vi "Keithley24XX_SR830_LakeShore336_I-Vg_Measurement.vi"() -> ()   [LabVIEW 2018]
uses:
  <instrlib>/Lake Shore 336/Public/Data/Sensor Data (Single Reading).vi
  <instrlib>/Stanford Research 830/Public/Data/Read (All Parameters).vi
  <instrlib>/Keithley 24XX/Public/Data/Read (Single Point).vi
  <instrlib>/Keithley 24XX/Keithley 24XX.lvlib
  <instrlib>/Stanford Research 830/Stanford Research 830.lvlib
  <instrlib>/Lake Shore 336/Lake Shore 336.lvlib
panel:
  in  "Loop Delay / Meas. Time (s)":dbl=1.0 format="%#_13g"
  out "Gate\nVoltage":sgl
  out "Status":sgl
  out "Leakage \nCurrent":sgl
  in  "Temp Vs Time":enum32{"XY Graph", "Waveform (Time)"}(tab)
  out "Temp vs Time : XYGraph":cluster{"Y":dbl[], "Y":dbl[]}[](graph)
  out "Temp vs Time : TimeGraph":cluster{i32, "Sensor Data":dbl}[](graph)
  in  "Data Source (0:Kelvin)":u16(ring) items=["Kelvin", "Celsius", "Sensor Units"]
  in  "Input (0:A)":u16(ring) items=["A", "B", "C", "D"]
  in  "Serial Configuration 2":T1={"Baud Rate"=57600, "Parity"=1, "Data Bits"=7, "Stop Bits"=10, "Flow Control"=0} {"Flow Control" items=["None", "XON/XOFF", "RTS/CTS", "XON/XOFF & RTS/CTS", "DTR/DSR", "XON/XOFF & DTR/DSR"]; "Stop Bits" items=["1.0"=10, "1.5"=15, "2.0"=20]; "Data Bits" items=["7"=7, "8"=8]; "Parity" items=["None", "Odd", "Even", "Mark", "Space"]; "Baud Rate" items=["300"=300, "600"=600, "1200"=1200, "2400"=2400, "4800"=4800, "9600"=9600, "19200"=19200, "38400"=38400, "57600"=57600]}
  in  "LakeShore 336 esource name":refnum<visa-resource-name>="GPIB0::12::INSTR"
  out "dup path":path
  in  "<File Name>.txt (Don't add extension)":string
  in  "Data Save Path:":path=path "C:/Users/labpc/Documents/ProbeStation Users Data"
  in  "I_leak vs Vg":enum32{"XY Graph", "Waveform (Time)"}(tab)
  out "I_leak vs Vg : XYGraph":cluster{"Y":dbl[], "Y":dbl[]}[](graph)
  out "I_leak vs Vg : TimeGraph":cluster{dbl, "Current":sgl}[](graph)
  in  "Gate Voltage\nInitial (V)":dbl
  out "Gate Voltage\nTraversal Direction":enum16{"Upward", "Downward"}(ring)
  in  "Gate Voltage \nStep Size (V)":dbl=0.1
  in  "High Gate \nVoltage (V)":dbl
  in  "Low Gate \nVoltage (V)":dbl
  in  "stop":bool
  out "Max/Min(-) \nGate Voltage (V)":dbl=80.0
  out "Compliance\n Level (A)":dbl=0.1
  in  "Theta vs Vg":enum32{"XY Graph", "Waveform (Time)"}(tab)
  out "Theta vs Vg : XYGraph":cluster{"Y":dbl[], "Y":dbl[]}[](graph)
  out "Theta vs Vg : TimeGraph":cluster{dbl, "Theta-Value":dbl}[](graph)
  in  "I vs Vg":enum32{"XY Graph", "Waveform (Time)"}(tab)
  out "Current vs Vg : XYGraph":cluster{"Y":dbl[], "Y":dbl[]}[](graph)
  out "I vs Vg : TimeGraph":cluster{dbl, dbl}[](graph)
  in  "Sensitivity (Initial Value)":i16(ring)=24 items=["Auto Gain"=-1, "2 nV/fA"=0, "5 nV/fA"=1, "10 nV/fA"=2, "20 nV/fA"=3, "50 nV/fA"=4, "100 nV/fA"=5, "200 nV/fA"=6, "500 nV/fA"=7, "1 uV/pA"=8, "2 uV/pA"=9, "5 uV/pA"=10, "10 uV/pA"=11, "20 uV/pA"=12, "50 uV/pA"=13, "100 uV/pA"=14, "200 uV/pA"=15, "500 uV/pA"=16, "1 mV/nA"=17, "2 mV/nA"=18, "5 mV/nA"=19, "10 mV/nA"=20, "20 mV/nA"=21, "50 mV/nA"=22, "100 mV/nA"=23, "200 mV/nA"=24, "500 mV/mA"=25, "1 V/uA"=26]
  in  "Dynamic Reserve (-1 = Auto)":i16(ring)=1 items=["Auto Reserve"=-1, "High Reserve"=0, "Normal"=1, "Low Noise"=2]
  in  "Input Connection (0: Single-Ended Voltage)":u16(ring)=2 items=["Single-Ended Voltage", "Differential Voltage", "1 MOhm Current Gain", "100 MOhm Current Gain"]
  out "Input Coupling (0: AC)":u16(ring) items=["AC", "DC"]
  in  "Time Constant (8: 100ms)":u16(ring)=9 items=["10 us", "30 us", "100 us", "300 us", "1 ms", "3 ms", "10 ms", "30 ms", "100 ms", "300 ms", "1 s", "3 s", "10 s", "30 s", "100 s", "300 s", "1 ks", "3 ks", "10 ks", "30 ks"]
  in  "SR830 VISA resource name":refnum<visa-resource-name>="GPIB0::10::INSTR"
  in  "Trigger Source (0: Internal)":u16(ring) items=["Internal", "External"]
  out "Manual Phase (0 Degree)":dbl
  out "Detection Harmonic Number":dbl=1.0
  out "External Reference Trigger (0: Sine Zero Crossing)":u16(ring) items=["Sine Zero Crossing", "TTL Rising Edge", "TTL Falling Edge"]
  in  "Internal Reference Frequency (1000 Hz)":dbl=7.6
  in  "Reference Source (1: Internal)":u16(ring)=1 items=["External", "Internal"]
  in  "Sine Output Amplitude (V)":dbl=1.0
  in  "Serial Configuration":T1={"Baud Rate"=9600, "Parity"=0, "Data Bits"=8, "Stop Bits"=10, "Flow Control"=0} {"Flow Control" items=["None", "XON/XOFF", "RTS/CTS", "XON/XOFF & RTS/CTS", "DTR/DSR", "XON/XOFF & DTR/DSR"]; "Stop Bits" items=["1.0"=10, "1.5"=15, "2.0"=20]; "Data Bits" items=["7"=7, "8"=8]; "Parity" items=["None", "Odd", "Even", "Mark", "Space"]; "Baud Rate" items=["300"=300, "600"=600, "1200"=1200, "2400"=2400, "4800"=4800, "9600"=9600, "19200"=19200]}
  in  "Keithley24XX VISA resource name":refnum<visa-resource-name>="GPIB0::21::INSTR" caption="Keithley 24XX VISA resource name"
  # "Lake Shore 336 Temp Contr."
  # "SR830 Lock In Amplifier"
  # "MAKE SURE THE SOURCE METER IS ON TO ENSURE NO UNINTENDED JUMPS. PROGRAM WILL KEEP SOURCE METER ON ONCE RUN."
  # "Keithley 2400 SourceMeter"
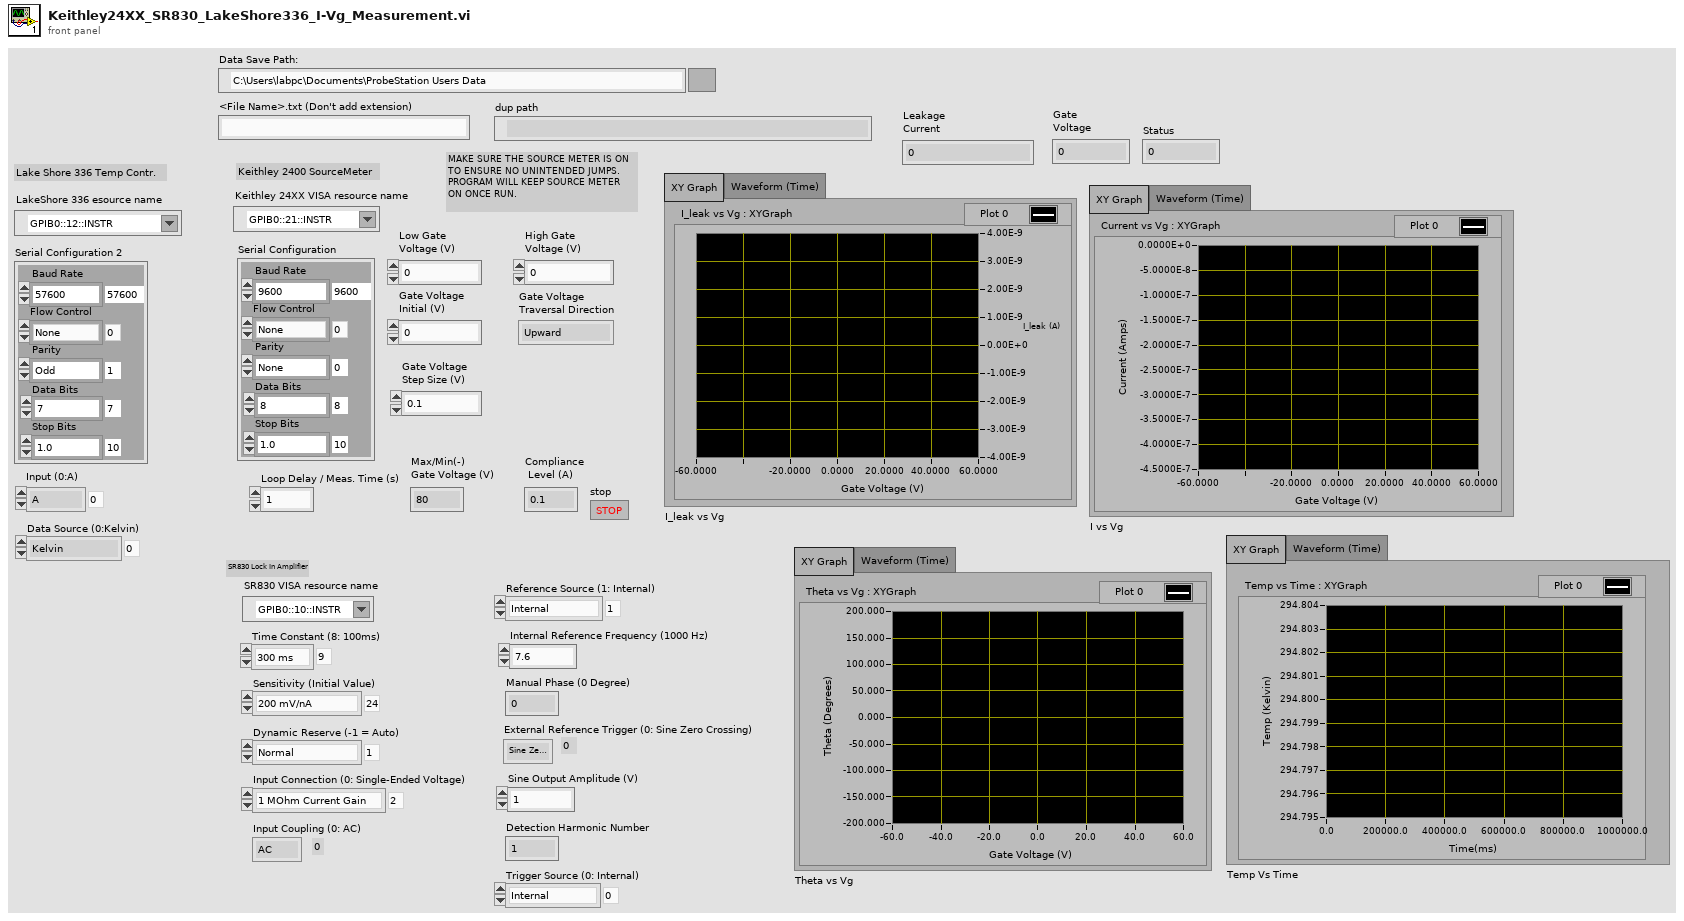
[diagram p1: front panel]
types:
  T1 = cluster{"Baud Rate":u32, "Parity":u16, "Data Bits":u16, "Stop Bits":u16, "Flow Control":u16}
  T2 = enum16{"open", "replace", "create", "open or create", "replace or create", "replace or create with confirmation"}
  T3 = cluster{"X-Value":dbl, "Y-Value":dbl, "R-Value":dbl, "Theta-Value":dbl, "Aux In 1 Value":dbl, "Aux In 2 Value":dbl, "Aux In 3 Value":dbl, "Aux In 4 Value":dbl, "Reference Frequency":dbl, "Channel 1 Display":dbl, "Channel 2 Display":dbl}
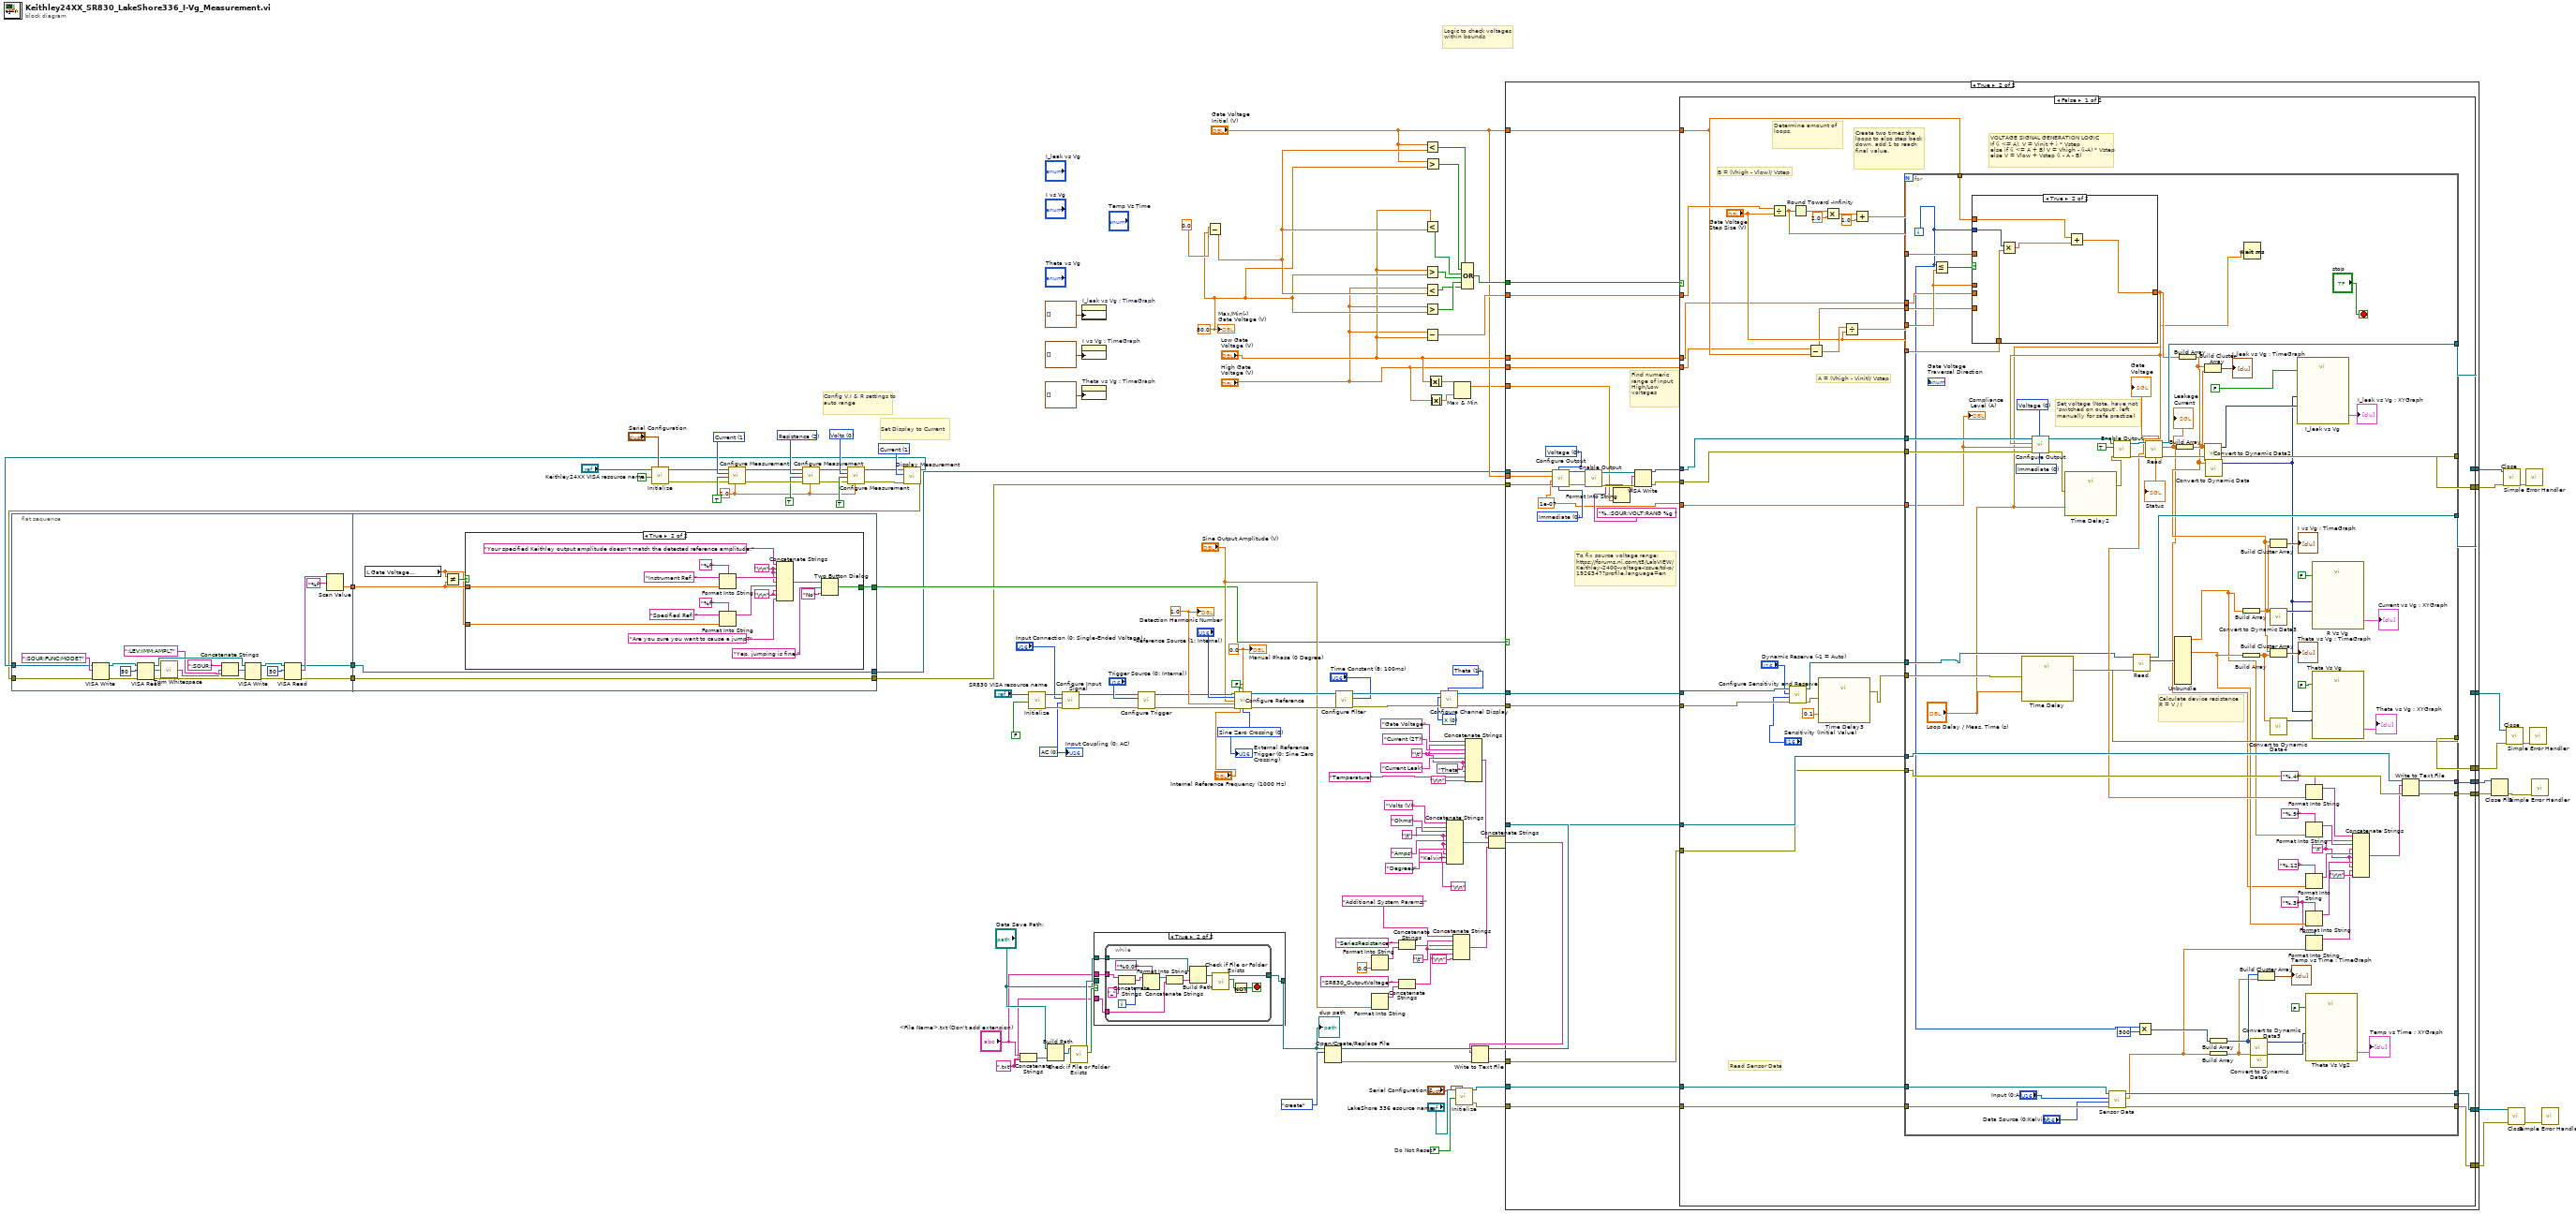
[diagram p0: block diagram]
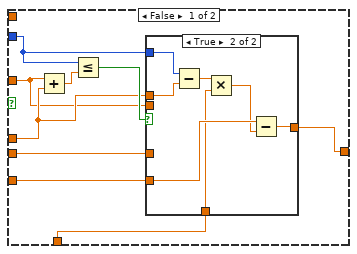
[diagram p3: hidden frame]
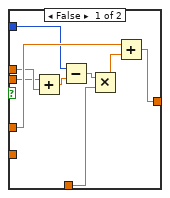
[diagram p4: hidden frame]
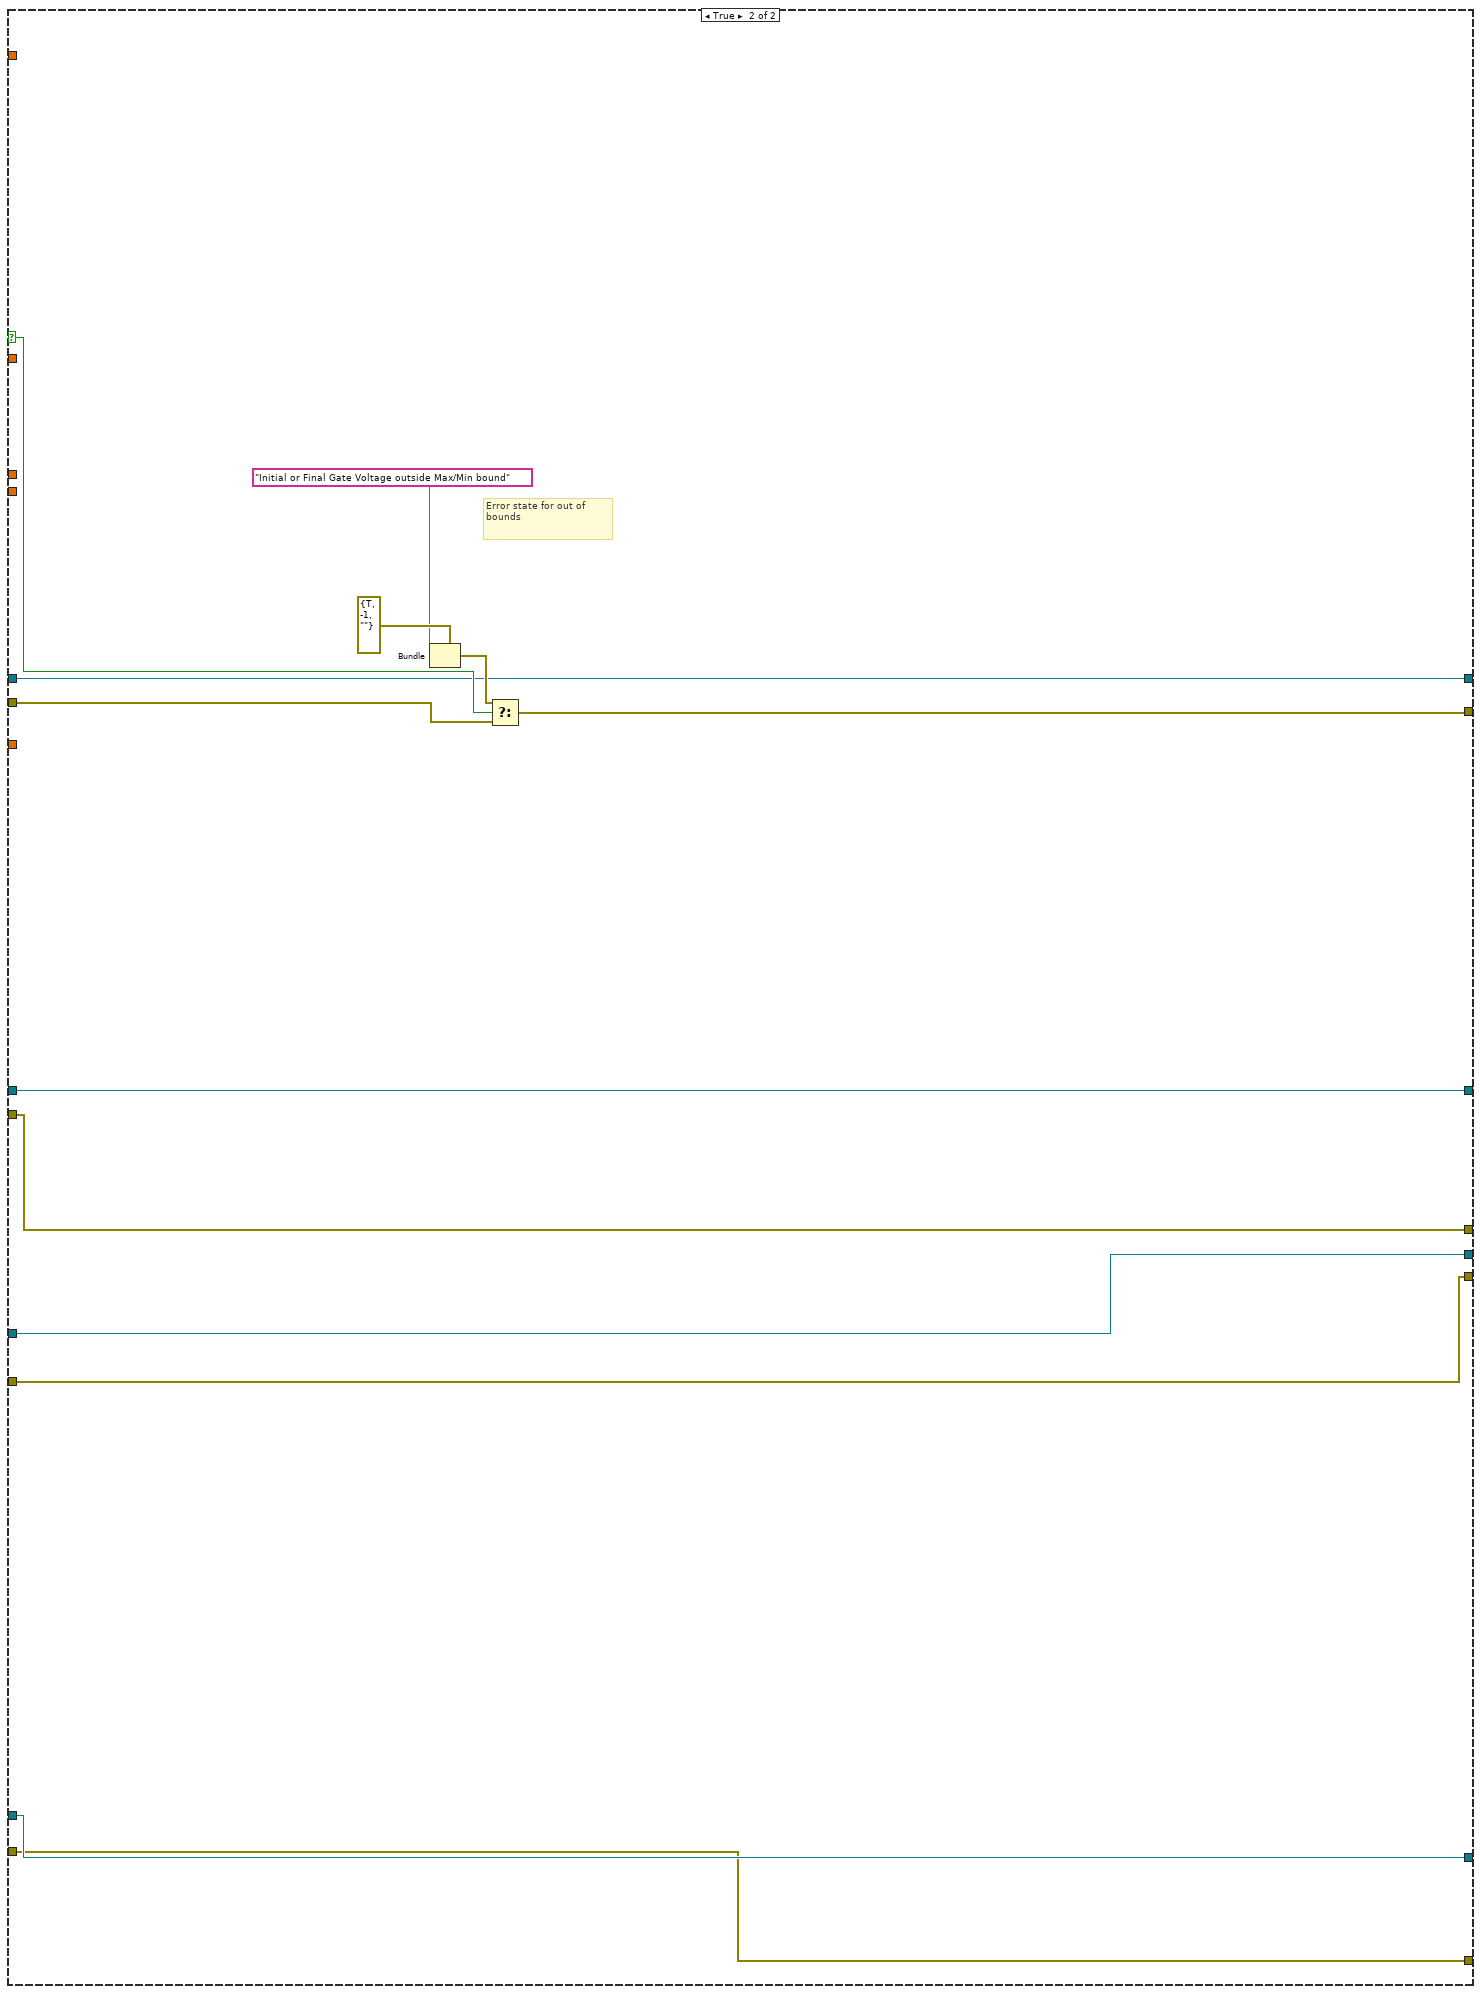
[diagram p5: hidden frame]
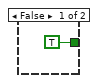
[diagram p6: hidden frame]
diagram:
  w28 = FALSE  # Do Not Reset
  w34 = "\t"
  w17 = "\t"
  w19 = "\t"
  w61 = ".txt"
  w68 = 1.0 ("Manual Range (1.0)")
  w91 = 0.0 ("Manual Phase (0 Degree)")
  w92 = 1.0 ("Detection Harmonic Number (1)")
  w93 = u16 0 items=["Sine Zero Crossing", "TTL Rising Edge", "TTL Falling Edge"] ("External Reference Trigger (0: Sine Zero Crossing)")
  w97 = u16 0 items=["AC", "DC"] ("Input Coupling (0: AC)")
  w80 = u16 0 items=["X", "R", "X Noise", "Aux In 1", "Aux In 2"] ("Channel 1 Display (0: X)")
  w107 = u16 1 items=["Y", "Theta", "Y Noise", "Aux In 3", "Aux In 4"] ("Channel 2 Display  (0: Y)")
  w112 = u16 1 items=["Voltage", "Current", "Resistance"] ("Displayed Measurement (0: Voltage)")
  w121 = u16 2 items=["Volts", "Current", "Resistance"] ("Function (0: Volts)")
  w125 = u16 1 items=["Volts", "Current", "Resistance"] ("Function (0: Volts)")
  w69 = 80.0
  w131 = u16 0 items=["Volts", "Current", "Resistance"] ("Function (0: Volts)")
  # "Logic to check voltages within bounds"
  # "Set Display to Current"
  # "Config V,I & R settings to auto range"
  n1 = flat-sequence {
    tunnel: [w135] -> w11
    tunnel: [w136] -> w10
    tunnel: [w137] -> w9
    tunnel: w8 -> [w134]
    tunnel: w7 -> [w133]
    tunnel: w11 -> [w156]
    tunnel: w10 -> [w155]
    tunnel: w9 -> [w159]
    tunnel: [w156] -> w3
    tunnel: [w155] -> w5
    tunnel: [w154] -> w6
    frame #0 {
      n2 = VISA Write(VISA resource name=w134, write buffer=":SOUR:FUNC:MODE?", error in (no error)=w133) -> (VISA resource name out=w150:refnum<visa-resource-name>, error out=w153:errorcluster)  [unwired: 1 out]
      n3 = VISA Read(VISA resource name=w150, byte count=u32 50, error in (no error)=w153) -> (VISA resource name out=w145:refnum<visa-resource-name>, read buffer=w139:string, error out=w146:errorcluster)  [unwired: 1 out]
      n4 = call <vilib>:"Trim Whitespace.vi"("string"=w139) -> ("trimmed string"=w138:string)  [unwired: 1 in]
      n5 = Concatenate Strings(":SOUR:" ("string"), w138, ":LEV:IMM:AMPL?" ("string")) -> (w142:string)
      n6 = VISA Write(VISA resource name=w145, write buffer=w142, error in (no error)=w146) -> (VISA resource name out=w147:refnum<visa-resource-name>, error out=w149:errorcluster)  [unwired: 1 out]
      n7 = VISA Read(VISA resource name=w147, byte count=u32 50, error in (no error)=w149) -> (VISA resource name out=w135:refnum<visa-resource-name>, read buffer=w140:string, error out=w136:errorcluster)  [unwired: 1 out]
      n8 = Scan Value(string=w140, format string="%f") -> (value=w137:dbl)  [unwired: 1 in, 1 out]
    }
    frame #1 {
      n9 = local read "Gate Voltage\nInitial (V)"() -> (w157:dbl)
      n10 = Not Equal?(x=w157, y=w159) -> (x != y?=w158:bool)
      n11 = case shown="True" w158 {
        tunnel: [TRUE ("T button?") w167] -> w154
        tunnel: w159 -> [_ w162]
        tunnel: w157 -> [_ w161]
        frame False {
        }
        frame True {
          w165 = "\r\n"
          w163 = "\r\n"
          n12 = Format Into String(format string="%f", initial string="Instrument Ref: ", w162) -> (resulting string=w169:string)  [unwired: 1 in, 1 out]
          n13 = Format Into String(format string="%f", initial string="Specified Ref: ", w161) -> (resulting string=w168:string)  [unwired: 1 in, 1 out]
          n14 = Concatenate Strings("Your specified Keithley output amplitude doesn't match the detected reference amplitude." ("message"), w163, w163, w169, w163, w168, w165, w165, "Are you sure you want to cause a jump?" ("string")) -> (w174:string)
          n15 = Two Button Dialog(message=w174, 1:"No" ("F button name (\"Cancel\")"), 2:"Yep, jumping is fine." ("T button name (\"OK\")")) -> (T button?=w167:bool)
        }
      }
    }
  }
  n16 = call <instrlib>:"Initialize.vi"("Serial Configuration"="Serial Configuration", "Reset (True)"=FALSE, "VISA resource name"="Keithley24XX VISA resource name") -> ("error out"=w116:errorcluster, "VISA resource name out"=w117:refnum<visa-resource-name>)  [unwired: 7 in]
  n17 = call <instrlib>:"Configure Measurement.vi"("Manual Range (1.0)"=w68, "error in (no error)"=w116, "Enable Auto Range (T:Enable)"=TRUE, "Function (0: Volts)"=w125, "VISA resource name"=w117) -> ("error out"=w123:errorcluster, "VISA resource name out"=w118:refnum<visa-resource-name>)  [unwired: 5 in]
  n18 = call <instrlib>:"Configure Measurement.vi"("Manual Range (1.0)"=w68, "error in (no error)"=w123, "Enable Auto Range (T:Enable)"=TRUE, "Function (0: Volts)"=w121, "VISA resource name"=w118) -> ("error out"=w120:errorcluster, "VISA resource name out"=w119:refnum<visa-resource-name>)  [unwired: 5 in]
  n19 = call <instrlib>:"Configure Measurement.vi"("Manual Range (1.0)"=w68, "error in (no error)"=w120, "Enable Auto Range (T:Enable)"=TRUE, "Function (0: Volts)"=w131, "VISA resource name"=w119) -> ("error out"=w110:errorcluster, "VISA resource name out"=w111:refnum<visa-resource-name>)  [unwired: 5 in]
  n20 = call <instrlib>:"Display Measurement.vi"("error in (no error)"=w110, "Displayed Measurement (0: Voltage)"=w112, "VISA resource name"=w111) -> ("error out"=w7:errorcluster, "VISA resource name out"=w8:refnum<visa-resource-name>)  [unwired: 7 in]
  n21 = Concatenate Strings("<File Name>.txt (Don't add extension)", w61) -> (w67:string)
  n22 = call <instrlib>:"Initialize.vi"("Reset (True)"=FALSE, "VISA resource name"="SR830 VISA resource name") -> ("error out"=w104:errorcluster, "VISA resource name out"=w105:refnum<visa-resource-name>)  [unwired: 8 in]
  n23 = Build Path(base path="Data Save Path:", name or relative path=w67) -> (appended path=w66:path)
  n24 = call <instrlib>:"Configure Input Signal.vi"("error in (no error)"=w104, "Input Coupling (0: AC)"=w97, "Input Connection (0: Single-Ended Voltage)"="Input Connection (0: Single-Ended Voltage)", "VISA resource name"=w105) -> ("error out"=w88:errorcluster, "VISA resource name out"=w89:refnum<visa-resource-name>)  [unwired: 6 in]
  n25 = call <vilib>:"Check if File or Folder Exists.vi"("path"=w66) -> ("file or folder exists?"=w65:bool, "dup path"=w64:path)  [unwired: 8 in, 1 out]
  n26 = property on="I_leak vs Vg : TimeGraph" class="WFChart (strict)"("History Data"=cluster{dbl, "Current":sgl}[] []) -> ()  [unwired: 2 in, 2 out]
  n27 = property on="I vs Vg : TimeGraph" class="WFChart (strict)"("History Data"=cluster{dbl, dbl}[] []) -> ()  [unwired: 2 in, 2 out]
  n28 = property on="Theta vs Vg : TimeGraph" class="WFChart (strict)"("History Data"=cluster{dbl, "Theta-Value":dbl}[] []) -> ()  [unwired: 2 in, 2 out]
  n29 = case shown="True" w65 {
    tunnel: [w177 w178] -> w58
    tunnel: w64 -> [w177 _]
    tunnel: "Data Save Path:" -> [_ w179]
    tunnel: "<File Name>.txt (Don't add extension)" -> [_ w181]
    tunnel: w61 -> [_ w180]
    frame False {
    }
    frame True {
      n30 = while {
        tunnel: w181 -> [w184]
        tunnel: w180 -> [w189]
        tunnel: w179 -> [w187]
        tunnel: [w185] -> w178
        i -> [w191]
        stop <- w193 stop-if-true
        n31 = Concatenate Strings(w184, "_" ("string")) -> (w183:string)
        n32 = Format Into String(format string="%0.0f", initial string=w183, w191) -> (resulting string=w190:string)  [unwired: 1 in, 1 out]
        n33 = Concatenate Strings(w190, w189) -> (w188:string)
        n34 = Build Path(base path=w187, name or relative path=w188) -> (appended path=w186:path)
        n35 = call <vilib>:"Check if File or Folder Exists.vi"("path"=w186) -> ("file or folder exists?"=w194:bool, "dup path"=w185:path)  [unwired: 8 in, 1 out]
        n36 = Not(x=w194) -> (.not. x?=w193:bool)
      }
    }
  }
  "dup path" <- w58
  n37 = call <instrlib>:"Configure Trigger.vi"("error in (no error)"=w88, "Trigger Source (0: Internal)"="Trigger Source (0: Internal)", "VISA resource name"=w89) -> ("error out"=w86:errorcluster, "VISA resource name out"=w87:refnum<visa-resource-name>)  [unwired: 7 in]
  n38 = Subtract(x=0.0, y=w69) -> (x-y=w74:dbl)
  n39 = call <instrlib>:"Configure Reference.vi"("VISA resource name"=w87, "Auto Phase (T: Enabled)"=FALSE, "Manual Phase (0 Degree)"=w91, "Reference Source (1: Internal)"="Reference Source (1: Internal)", "Sine Output Amplitude (1 V)"="Sine Output Amplitude (V)", "Detection Harmonic Number (1)"=w92, "error in (no error)"=w86, "Internal Reference Frequency (1000 Hz)"="Internal Reference Frequency (1000 Hz)", "External Reference Trigger (0: Sine Zero Crossing)"=w93) -> ("VISA resource name out"=w94:refnum<visa-resource-name>, "error out"=w95:errorcluster)  [unwired: 5 in]
  n40 = Open/Create/Replace File(file path (use dialog)=w58, operation (0:open)=T2."create") -> (refnum out=w59:refnum<file>, error out=w57:errorcluster)  [unwired: 4 in, 1 out]
  n41 = call <instrlib>:"Configure Filter.vi"("error in (no error)"=w95, "Time Constant (8: 100ms)"="Time Constant (8: 100ms)", "VISA resource name"=w94) -> ("error out"=w114:errorcluster, "VISA resource name out"=w113:refnum<visa-resource-name>)  [unwired: 7 in]
  n42 = Format Into String(0.0 ("input 1")) -> (resulting string=w51:string)  [unwired: 3 in, 1 out]
  n43 = Format Into String("Sine Output Amplitude (V)") -> (resulting string=w50:string)  [unwired: 3 in, 1 out]
  n44 = Concatenate Strings("SeriesResistance:" ("string"), w51) -> (w33:string)
  n45 = Concatenate Strings("SR830_OutputVoltage:" ("string"), w50) -> (w32:string)
  n46 = Less?(x="Gate Voltage\nInitial (V)", y=w74) -> (x < y?=w72:bool)
  n47 = Less?(x="Low Gate \nVoltage (V)", y=w74) -> (x < y?=w78:bool)
  n48 = Greater?(x="Low Gate \nVoltage (V)", y=w69) -> (0:w77:bool)
  n49 = Less?(x="High Gate \nVoltage (V)", y=w74) -> (x < y?=w75:bool)
  n50 = Greater?(x="High Gate \nVoltage (V)", y=w69) -> (0:w76:bool)
  n51 = Subtract(x="High Gate \nVoltage (V)", y="Low Gate \nVoltage (V)") -> (x-y=w70:dbl)
  n52 = Greater?(x="Gate Voltage\nInitial (V)", y=w69) -> (0:w73:bool)
  n53 = Absolute Value(x="Low Gate \nVoltage (V)") -> (abs(x)=w15:dbl)
  n54 = Absolute Value(x="High Gate \nVoltage (V)") -> (abs(x)=w14:dbl)
  n55 = call <instrlib>:"Configure Channel Display.vi"("Channel 2 Display  (0: Y)"=w107, "error in (no error)"=w114, "Channel 1 Display (0: X)"=w80, "VISA resource name"=w113) -> ("error out"=w102:errorcluster, "VISA resource name out"=w103:refnum<visa-resource-name>)  [unwired: 6 in]
  n56 = Concatenate Strings("Volts (V)" ("string"), w17, "Ohms" ("string"), w17, "Amps" ("string"), w17, "Degrees" ("string"), w17, "Kelvin" ("string"), "\r\n") -> (w45:string)
  n57 = Concatenate Strings("Additional System Params:" ("string"), w34, w33, w34, w32, "\r\n") -> (w35:string)
  n58 = Max & Min(x=w15, y=w14) -> (max(x,y)=w2:dbl)  [unwired: 1 out]
  n59 = call <instrlib>:"Initialize.vi"("Serial Configuration"="Serial Configuration 2", "Reset (True)"=w28, "VISA resource name"="LakeShore 336 esource name") -> ("error out"=w23:errorcluster, "VISA resource name out"=w22:refnum<visa-resource-name>)  [unwired: 7 in]
  n60 = Compound Arithmetic op=OR(w72, w73, w78, w77, w76, w75) -> (w71:bool)
  n61 = Concatenate Strings("Gate Voltage" ("string"), w19, "Current (2T)" ("string"), w19, "Current Leak" ("string"), w19, "Theta" ("string"), w19, "Temperature" ("string"), "\r\n") -> (w46:string)
  n62 = Concatenate Strings(w46, w45, w35) -> (w30:string)
  n63 = Write to Text File(file (use dialog)=w59, text=w30, error in=w57) -> (refnum out=w55:refnum<file>, error out=w54:errorcluster)  [unwired: 1 in, 1 out]
  n64 = case shown="True" w6 {
    tunnel: [w202 w236] -> w129
    tunnel: [w201 w235] -> w128
    tunnel: w103 -> [w200 w234]
    tunnel: w102 -> [w199 w233]
    tunnel: [w200 w232] -> w101
    tunnel: [w199 w231] -> w100
    tunnel: w71 -> [_ w230]
    tunnel: w70 -> [_ w229]
    tunnel: w55 -> [w198 w228]
    tunnel: w54 -> [w197 w227]
    tunnel: [w198 w226] -> w53
    tunnel: [w197 w225] -> w52
    tunnel: [w195 w224] -> w25
    tunnel: [w196 w223] -> w24
    tunnel: w23 -> [w195 w222]
    tunnel: w22 -> [w196 w221]
    tunnel: "Low Gate \nVoltage (V)" -> [_ w220]
    tunnel: "High Gate \nVoltage (V)" -> [_ w219]
    tunnel: "Gate Voltage\nInitial (V)" -> [_ w218]
    tunnel: w5 -> [w201 w210]
    tunnel: "Gate Voltage\nInitial (V)" -> [_ w209]
    tunnel: w3 -> [w202 w208]
    tunnel: w2 -> [_ w206]
    frame False {
    }
    frame True {
      w212 = u16 0 items=["Immediate", "Triggered"] ("Output Type  (0: Immediate)")
      w205 = 1e-07 ("Compliance  Level (0.1)")
      w211 = u16 0 items=["Voltage", "Current"] ("Source Mode  (0: Voltage)")
      # "Find numeric range of input High/Low voltages"
      # "To fix source voltage range:\nhttps://forums.ni.com/t5/LabVIEW/Keithley-2400-voltage-Issue/td-p/1926347?profile.language=en"
      n65 = call <instrlib>:"Configure Output.vi"("Output Type  (0: Immediate)"=w212, "Source Mode  (0: Voltage)"=w211, "error in (no error)"=w210, "Compliance  Level (0.1)"=w205, "Output Level (0)"=w209, "VISA resource name"=w208) -> ("error out"=w217:errorcluster, "VISA resource name out"=w216:refnum<visa-resource-name>)  [unwired: 4 in]
      n66 = call <instrlib>:"Enable Output.vi"("error in (no error)"=w217, "VISA resource name"=w216) -> ("error out"=w215:errorcluster, "VISA resource name out"=w214:refnum<visa-resource-name>)  [unwired: 8 in]
      n67 = Format Into String(format string="%.;SOUR:VOLT:RANG %g ", w206) -> (resulting string=w213:string)  [unwired: 2 in, 1 out]
      n68 = VISA Write(VISA resource name=w214, write buffer=w213, error in (no error)=w215) -> (VISA resource name out=w203:refnum<visa-resource-name>, error out=w204:errorcluster)  [unwired: 1 out]
      n69 = case shown="False" w230 {
        selector: w230 -> [_ w399]
        tunnel: w204 -> [w272 w398]
        tunnel: w203 -> [w238 w393]
        tunnel: [w271 w393] -> w236
        tunnel: [w270 w394] -> w235
        tunnel: w234 -> [w265 w392]
        tunnel: w233 -> [w266 w391]
        tunnel: [w268 w392] -> w232
        tunnel: [w267 w391] -> w231
        tunnel: w229 -> [w258 _]
        tunnel: w220 -> [w251 _]
        tunnel: w219 -> [w252 _]
        tunnel: w218 -> [w254 _]
        tunnel: w228 -> [w247 w390]
        tunnel: w227 -> [w246 w389]
        tunnel: [w245 w390] -> w226
        tunnel: [w244 w389] -> w225
        tunnel: [w240 w387] -> w224
        tunnel: [w239 w388] -> w223
        tunnel: w222 -> [w242 w387]
        tunnel: w221 -> [w241 w388]
        tunnel: w205 -> [w237 _]
        frame False {
          # "Read Sensor Data"
          # "VOLTAGE SIGNAL GENERATION LOGIC\nIf (i <= A), V = Vinit + i * Vstep\nelse if (i <= A + B) V = Vhigh - (i-A) * Vstep\nelse V = Vlow + Vstep (i - A - B)"
          # "B = (Vhigh - Vlow)/ Vstep"
          # "A = (Vhigh - Vinit)/ Vstep"
          # "Create two times the loops to also step back down, add 1 to reach final value."
          # "Determine amount of loops,"
          n70 = Divide(x=w258, y="Gate Voltage \nStep Size (V)") -> (x/y=w253:dbl)
          n71 = call <instrlib>:"Configure Sensitivity and Reserve.vi"("error in (no error)"=w266, "Sensitivity (-1: Auto gain)"="Sensitivity (Initial Value)", "Dynamic Reserve (-1: Auto Reserve)"="Dynamic Reserve (-1 = Auto)", "VISA resource name"=w265) -> ("error out"=w249:errorcluster, "VISA resource name out"=w264:refnum<visa-resource-name>)  [unwired: 6 in]
          n72 = Round Toward -Infinity(1:w253) -> (0:w261:dbl)
          n73 = Subtract(x=w252, y=w254) -> (x-y=w257:dbl)
          n74 = call "Time Delay3"("error in (no error)"=w249, "Delay Time (s)"=0.1) -> ("error out"=w250:errorcluster)  [unwired: 9 in]
          n75 = Multiply(x=w261, y=2.0) -> (x*y=w260:dbl)
          n76 = Divide(x=w257, y="Gate Voltage \nStep Size (V)") -> (x/y=w255:dbl)
          n77 = Add(x=w260, y=1.0) -> (x+y=w259:dbl)
          n78 = for {
            N: w259 -> [_]
            tunnel: w238 -> [w353]
            tunnel: w272 -> [w320]
            tunnel: [w356] -> w271
            tunnel: [w355] -> w270
            tunnel: [w346] -> w268
            tunnel: [w347] -> w267
            tunnel: w264 -> [w302]
            tunnel: w250 -> [w303]
            tunnel: "Gate Voltage \nStep Size (V)" -> [w326]
            tunnel: w255 -> [w324]
            tunnel: w254 -> [w327]
            tunnel: w253 -> [w325]
            tunnel: w252 -> [w323]
            tunnel: w251 -> [w322]
            tunnel: w247 -> [w317]
            tunnel: w246 -> [w316]
            tunnel: [w315] -> w245
            tunnel: [w314] -> w244
            tunnel: w242 -> [w295]
            tunnel: w241 -> [w294]
            tunnel: [w293] -> w240
            tunnel: [w292] -> w239
            tunnel: w237 -> [w275]
            i -> [w286]
            stop <- "stop" stop-if-true
            w283 = "%.3f" ("format string")
            w280 = "\t"
            w321 = u16 0 items=["Immediate", "Triggered"] ("Output Type  (0: Immediate)")
            w349 = u16 0 items=["Voltage", "Current"] ("Source Mode  (0: Voltage)")
            # "Calculate device resistance\nR = V / I"
            # "Set voltage (Note, have not 'switched on output', left manually for safe practise)"
            n79 = Less Or Equal?(x=w286, y=w324) -> (x <= y?=w328:bool)
            n80 = case shown="True" w328 {
              tunnel: [w363 w382] -> w308
              tunnel: w327 -> [_ w385]
              tunnel: w286 -> [w360 w386]
              tunnel: w326 -> [w361 w383]
              tunnel: w325 -> [w357 _]
              tunnel: w324 -> [w359 _]
              tunnel: w323 -> [w362 _]
              tunnel: w322 -> [w358 _]
              frame False {
                n81 = Add(x=w357, y=w359) -> (x+y=w364:dbl)
                n82 = Less Or Equal?(x=w360, y=w364) -> (x <= y?=w365:bool)
                n83 = case shown="True" w365 {
                  tunnel: [w371 w380] -> w363
                  tunnel: w362 -> [_ w381]
                  tunnel: w361 -> [w373 w378]
                  tunnel: w360 -> [w368 w377]
                  tunnel: w359 -> [w367 w376]
                  tunnel: w358 -> [w374 _]
                  tunnel: w357 -> [w366 _]
                  frame False {
                    n84 = Add(x=w366, y=w367) -> (x+y=w369:dbl)
                    n85 = Subtract(x=w368, y=w369) -> (x-y=w370:dbl)
                    n86 = Multiply(x=w370, y=w373) -> (x*y=w372:dbl)
                    n87 = Add(x=w374, y=w372) -> (x+y=w371:dbl)
                  }
                  frame True {
                    n88 = Subtract(x=w377, y=w376) -> (x-y=w379:dbl)
                    n89 = Multiply(x=w379, y=w378) -> (x*y=w375:dbl)
                    n90 = Subtract(x=w381, y=w375) -> (x-y=w380:dbl)
                  }
                }
              }
              frame True {
                n91 = Multiply(x=w386, y=w383) -> (x*y=w384:dbl)
                n92 = Add(x=w385, y=w384) -> (x+y=w382:dbl)
              }
            }
            n93 = call "Time Delay"("error in (no error)"=w303, "Delay Time (s)"="Loop Delay / Meas. Time (s)") -> ("error out"=w344:errorcluster)  [unwired: 9 in]
            n94 = call <instrlib>:"Configure Output.vi"("Output Type  (0: Immediate)"=w321, "Source Mode  (0: Voltage)"=w349, "error in (no error)"=w320, "Compliance  Level (0.1)"=w275, "Output Level (0)"=w308, "VISA resource name"=w353) -> ("error out"=w319:errorcluster, "VISA resource name out"=w352:refnum<visa-resource-name>)  [unwired: 4 in]
            n95 = call "Time Delay2"("error in (no error)"=w319, "Delay Time (s)"="Loop Delay / Meas. Time (s)") -> ("error out"=w318:errorcluster)  [unwired: 9 in]
            n96 = call-poly <instrlib>:"Sensor Data.vi"("error in (no error)"=w295, "Data Source (0:Kelvin)"="Data Source (0:Kelvin)", "Input (0:A)"="Input (0:A)", "VISA resource name"=w294) -> ("error out"=w293:errorcluster, "Sensor Data"=w282:dbl, "VISA resource name out"=w292:refnum<visa-resource-name>)  [unwired: 5 in]
            n97 = call <instrlib>:"Enable Output.vi"("error in (no error)"=w318, "Enable Output (T: Enable)"=TRUE, "VISA resource name"=w352) -> ("error out"=w351:errorcluster, "VISA resource name out"=w350:refnum<visa-resource-name>)  [unwired: 7 in]
            n98 = call-poly <instrlib>:"Read.vi"("error in (no error)"=w344, "VISA resource name"=w302) -> ("error out"=w347:errorcluster, "Parameter Values"=w345:T3, "VISA resource name out"=w346:refnum<visa-resource-name>)  [unwired: 7 in]
            n99 = Multiply(x=w286, y=500) -> (x*y=w284:i32)
            n100 = call-poly <instrlib>:"Read.vi"("VISA resource name"=w350, "error in (no error)"=w351) -> ("Voltage"=→"Gate\nVoltage":sgl, "VISA resource name out"=w356:refnum<visa-resource-name>, "Current"=w278:sgl, "Status"=→"Status":sgl, "error out"=w355:errorcluster)  [unwired: 7 in, 2 out]
            "Leakage \nCurrent" <- w278
            n101 = Unbundle(w345) -> ("X-Value"=w274:dbl, "Theta-Value"=w307:dbl)  [unwired: 9 out]
            n102 = Build Array(w278) -> (w341:sgl[])
            n103 = Build Array(w308) -> (w299:dbl[])
            n104 = Build Cluster Array(w299, w341) -> (→"I_leak vs Vg : TimeGraph":cluster{dbl, "Current":sgl}[])
            n105 = call "Convert to Dynamic Data2"("Array"=w341) -> ("Dynamic Data Type"=w340:dynamicdata)  [unwired: 3 in]
            n106 = call "Convert to Dynamic Data"("Array"=w299) -> ("Dynamic Data Type"=w298:dynamicdata)  [unwired: 3 in]
            n107 = Build Array(w284) -> (w296:i32[])
            n108 = Build Array(w282) -> (w288:dbl[])
            n109 = Build Array(w274) -> (w339:dbl[])
            n110 = Build Array(w307) -> (w337:dbl[])
            n111 = Wait (ms)(milliseconds to wait="Loop Delay / Meas. Time (s)") -> ()  [unwired: 1 out]
            n112 = call "Convert to Dynamic Data5"("Array"=w296) -> ("Dynamic Data Type"=w297:dynamicdata)  [unwired: 3 in]
            n113 = call "Convert to Dynamic Data6"("Array"=w288) -> ("Dynamic Data Type"=w289:dynamicdata)  [unwired: 3 in]
            n114 = Build Cluster Array(w296, w288) -> (→"Temp vs Time : TimeGraph":cluster{i32, "Sensor Data":dbl}[])
            n115 = Build Cluster Array(w299, w339) -> (→"I vs Vg : TimeGraph":cluster{dbl, "X-Value":dbl}[])
            n116 = call "Convert to Dynamic Data3"("Array"=w339) -> ("Dynamic Data Type"=w338:dynamicdata)  [unwired: 3 in]
            n117 = Build Cluster Array(w299, w337) -> (→"Theta vs Vg : TimeGraph":cluster{dbl, "Theta-Value":dbl}[])
            n118 = call "Convert to Dynamic Data4"("Array"=w337) -> ("Dynamic Data Type"=w336:dynamicdata)  [unwired: 3 in]
            n119 = call "I_leak vs Vg"("Reset"=FALSE, "Y Input"=w340, "X Input"=w298) -> ("XY Graph"=→"I_leak vs Vg : XYGraph":cluster{"X":dbl[], "Y":dbl[]}[])  [unwired: 7 in, 1 out]
            n120 = Format Into String(format string="%.4f", w308) -> (resulting string=w313:string)  [unwired: 2 in, 1 out]
            n121 = Format Into String(format string="%.9f", w274) -> (resulting string=w312:string)  [unwired: 2 in, 1 out]
            n122 = Format Into String(format string="%.12f", w278) -> (resulting string=w311:string)  [unwired: 2 in, 1 out]
            n123 = Format Into String(format string=w283, w307) -> (resulting string=w310:string)  [unwired: 2 in, 1 out]
            n124 = Format Into String(format string=w283, w282) -> (resulting string=w279:string)  [unwired: 2 in, 1 out]
            n125 = call "Theta Vs Vg2"("Reset"=FALSE, "Y Input"=w289, "X Input"=w297) -> ("XY Graph"=→"Temp vs Time : XYGraph":cluster{"X":dbl[], "Y":dbl[]}[])  [unwired: 7 in, 1 out]
            n126 = call "R Vs Vg"("Reset"=FALSE, "Y Input"=w338, "X Input"=w298) -> ("XY Graph"=→"Current vs Vg : XYGraph":cluster{"X":dbl[], "Y":dbl[]}[])  [unwired: 7 in, 1 out]
            n127 = call "Theta Vs Vg"("Reset"=FALSE, "Y Input"=w336, "X Input"=w298) -> ("XY Graph"=→"Theta vs Vg : XYGraph":cluster{"X":dbl[], "Y":dbl[]}[])  [unwired: 7 in, 1 out]
            n128 = Concatenate Strings(w313, w280, w312, w280, w311, w280, w310, w280, w279, "\r\n") -> (w309:string)
            n129 = Write to Text File(file (use dialog)=w317, text=w309, error in=w316) -> (refnum out=w315:refnum<file>, error out=w314:errorcluster)  [unwired: 1 in, 1 out]
            "Compliance\n Level (A)" <- w275
          }
        }
        frame True {
          # "Error state for out of bounds"
          n130 = Bundle(cluster=errorcluster {"status"=TRUE, "code"=-1, "source"=""} ("error constant"), "source"="Initial or Final Gate Voltage outside Max/Min bound") -> (w395:errorcluster)  [unwired: 2 in]
          n131 = Select(t=w395, s=w399, f=w398) -> (s? t:f=w394:errorcluster)
        }
      }
    }
  }
  n132 = Close File(refnum=w53, error in=w52) -> (error out=w56:errorcluster)  [unwired: 1 out]
  n133 = call <instrlib>:"Close.vi"("error in (no error)"=w128, "VISA resource name"=w129) -> ("error out"=w127:errorcluster)  [unwired: 9 in]
  n134 = call <instrlib>:"Close.vi"("error in (no error)"=w100, "VISA resource name"=w101) -> ("error out"=w115:errorcluster)  [unwired: 9 in]
  n135 = call <instrlib>:"Close.vi"("error in (no error)"=w25, "VISA resource name"=w24) -> ("error out"=w26:errorcluster)  [unwired: 9 in]
  n136 = call <vilib>:"Simple Error Handler.vi"("error in (no error)"=w127) -> ()  [unwired: 4 in, 5 out]
  n137 = call <vilib>:"Simple Error Handler.vi"("error in (no error)"=w115) -> ()  [unwired: 4 in, 5 out]
  n138 = call <vilib>:"Simple Error Handler.vi"("error in (no error)"=w56) -> ()  [unwired: 4 in, 5 out]
  n139 = call <vilib>:"Simple Error Handler.vi"("error in (no error)"=w26) -> ()  [unwired: 4 in, 5 out]
  "Max/Min(-) \nGate Voltage (V)" <- w69
  "Input Coupling (0: AC)" <- w97
  "External Reference Trigger (0: Sine Zero Crossing)" <- w93
  "Detection Harmonic Number" <- w92
  "Manual Phase (0 Degree)" <- w91
